vi "fgv_StimTrigFunct-Setup.vi"(0 "Function":enum16{"Intialize", "Write", "Read", "Clear"}(ring), 5 "Live stim.trig.enable":bool, 7 "Funct stim.trig.delay (sec)":dbl, 9 "Funct stim.trig.width (ms)":dbl, 11 "error in (no error)":errorcluster) -> (6 "Live stim.trig.enable":bool, 8 "Funct stim.trig.delay (sec)":dbl, 10 "Funct stim.trig.width (ms)":dbl, 15 "error out":errorcluster)   [LabVIEW 2017]
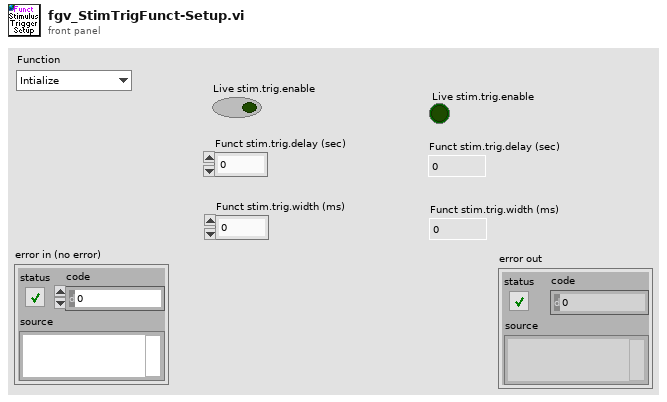
[diagram p1: front panel]
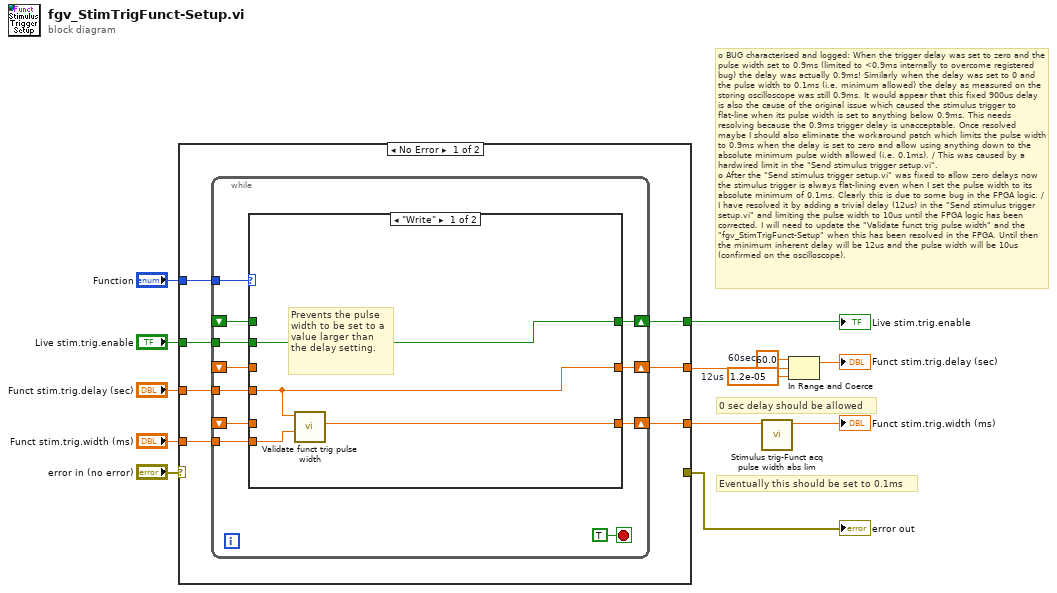
[diagram p0: block diagram]
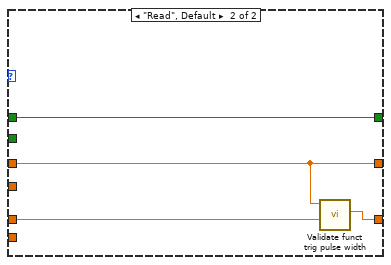
[diagram p2: hidden frame]
diagram:
  w6 = 60.0  # 60sec
  w7 = 1.2e-05  # 12us
  # "Eventually this should be set to 0.1ms"
  # "0 sec delay should be allowed"
  # "o\tBUG characterised and logged: When the trigger delay was set to zero and the pulse width set to 0.9ms (limited to <0.9ms internally to overcome registered bug) the delay was actually 0.9ms! Similarly when the delay was set to 0 and the pulse width to 0.1ms (i.e. minimum allowed) the delay as measured on the storing oscilloscope was still 0.9ms. It would appear that this fixed 900us delay is also the cause of the original issue which caused the stimulus trigger to flat-line when its pulse width is set to anything below 0.9ms. This needs resolving because the 0.9ms trigger delay is unacceptable. Once resolved maybe I should also eliminate the workaround patch which limits the pulse width to 0.9ms when the delay is set to zero and allow using anything down to the absolute minimum pulse width allowed (i.e. 0.1ms). / This was caused by a hardwired limit in the \"Send stimulus trigger setup.vi\".\no\tAfter the \"Send stimulus trigger setup.vi\" was fixed to allow zero delays now the stimulus trigger is always flat-lining even when I set the pulse width to its absolute minimum of 0.1ms. Clearly this is due to some bug in the FPGA logic. / I have resolved it by adding a trivial delay (12us) in the \"Send stimulus trigger setup.vi\" and limiting the pulse width to 10us until the FPGA logic has been corrected. I will need to update the \"Validate funct trig pulse width\" and the \"fgv_StimTrigFunct-Setup\" when this has been resolved in the FPGA. Until then the minimum inherent delay will be 12us and the pulse width will be 10us (confirmed on the oscilloscope)."
  n1 = case shown="No Error" "error in (no error)" {
    selector: "error in (no error)" -> [_ w43]
    tunnel: [_ w43] -> w2
    tunnel: "Function" -> [w20 _]
    tunnel: "Live stim.trig.enable" -> [w19 w42]
    tunnel: [w18 w42] -> w10
    tunnel: "Funct stim.trig.delay (sec)" -> [w17 w41]
    tunnel: [w16 w41] -> w5
    tunnel: "Funct stim.trig.width (ms)" -> [w15 w40]
    tunnel: [w14 w40] -> w1
    frame No Error {
      n2 = while {
        tunnel: w20 -> [w30]
        tunnel: w19 -> [w29]
        shift-right: [w28] -> w18
        shift-left: _ -> [w27]
        tunnel: w17 -> [w25]
        shift-right: [w26] -> w16
        shift-left: _ -> [w24]
        tunnel: w15 -> [w23]
        shift-right: [w22] -> w14
        shift-left: _ -> [w21]
        stop <- TRUE stop-if-true
        n3 = case shown="\"Write\"" w30 {
          tunnel: [w35 w39] -> w28
          tunnel: w29 -> [w35 _]
          tunnel: w27 -> [_ w39]
          tunnel: [w34 w38] -> w26
          tunnel: w25 -> [w34 _]
          tunnel: w24 -> [_ w38]
          tunnel: w23 -> [w33 _]
          tunnel: [w32 w36] -> w22
          tunnel: w21 -> [_ w37]
          frame "Write" {
            # "Prevents the pulse width to be set to a value larger than the delay setting."
            n4 = call "Validate funct trig pulse width.vi"("Requested trigger pulse width (ms)"=w33, "Trigger delay (sec)"=w34) -> ("functional acq. stimulus trigger pulse width (ms)"=w32:dbl)  [unwired: 9 in]
          }
          frame "Read", Default {
            n5 = call "Validate funct trig pulse width.vi"("Requested trigger pulse width (ms)"=w37, "Trigger delay (sec)"=w38) -> ("functional acq. stimulus trigger pulse width (ms)"=w36:dbl)  [unwired: 9 in]
          }
        }
      }
    }
    frame Error {
    }
  }
  "error out" <- w2
  "Live stim.trig.enable" <- w10
  n6 = call "Stimulus trig-Funct acq pulse width abs lim.vi"("Funct acq. stimulus trigger pulse width (ms)"=w1) -> ("Funct acq. stimulus trigger pulse width (ms)"=→"Funct stim.trig.width (ms)":dbl)  [unwired: 10 in]
  n7 = In Range and Coerce(upper limit=w6, x=w5, lower limit=w7) -> (coerced(x)=→"Funct stim.trig.delay (sec)":dbl)  [unwired: 1 out]
